vi "Stop Core.vi"(10 "final error code":i32 caption="code d'erreur final", 11 "Dual Fan in":refnum<class "Dual Fan.lvclass"> caption="Acteur en entrée") -> (3 "Dual Fan out":refnum<class "Dual Fan.lvclass"> caption="Acteur en sortie")   [LabVIEW 2015, in "Dual Fan.lvlib" / "Dual Fan.lvclass"]
doc: "(<B>Nom de fichier</B> : Actor Framework.lvlib:Actor.lvclass:Stop Core.vi)\n\nDéfinit ce que l'acteur fait avant de s'arrêter. Utilisez l'entrée <B>code d'erreur final</B> pour déterminer si l'acteur se ferme en réponse à une erreur.\n\nPar défaut, cette méthode ne fait rien. Une classe descendante peut la redéfinir pour configurer un comportement, tel que la fermeture des processus initialisés par l'acteur dans sa redéfinition de la méthode Noyau d'acteur."
uses:
  Dual Fan.lvclass
  Timed Loop Controller/Timed Loop Controller/Timed Loop Controller.lvclass
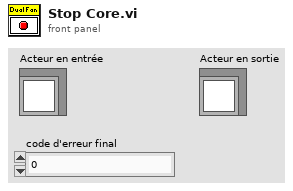
[diagram p1: front panel]
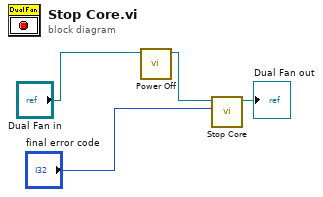
[diagram p0: block diagram]
diagram:
  n1 = call "Power Off.vi"("Dual Fan in"="Dual Fan in") -> ("Dual Fan out"=w1:refnum<class "Dual Fan.lvclass">)  [unwired: 9 in, 1 out]
  n2 = call-parent "Stop Core.vi"("final error code"="final error code", "Actor in"=w1) -> ("Actor out"=→"Dual Fan out":refnum<class "Dual Fan.lvclass">)  [unwired: 9 in]
